vi "Handle.vi"(7 "Event in":refnum<class "Event.lvclass">, 11 "Teardown State in":refnum<class "Teardown State.lvclass">) -> (2 "Destroy?":bool, 5 "Event out":refnum<class "Event.lvclass">)   [LabVIEW 2021, in "jettl.lvlib" / "Base Event.lvlib" / "State.lvlib" / "Teardown State.lvclass"]
uses:
  Teardown State.lvclass
  Event/Event.lvclass
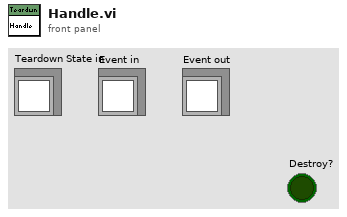
[diagram p1: front panel]
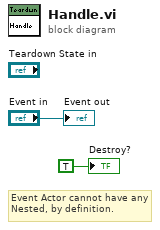
[diagram p0: block diagram]
diagram:
  # "Event Actor cannot have any Nested, by definition."
  "Destroy?" <- TRUE ("Destroy?")
  "Event out" <- "Event in"
